vi "Create.vi"(8 "error in (no error)":errorcluster) -> (0 "error out":errorcluster, 3 "BL-Retract-Cmd.lvclass":refnum<class "BL-Retract-Cmd.lvclass">)   [LabVIEW 2013, in "BL-Retract-Cmd.lvclass"]
uses:
  BL-Retract-Cmd.lvclass
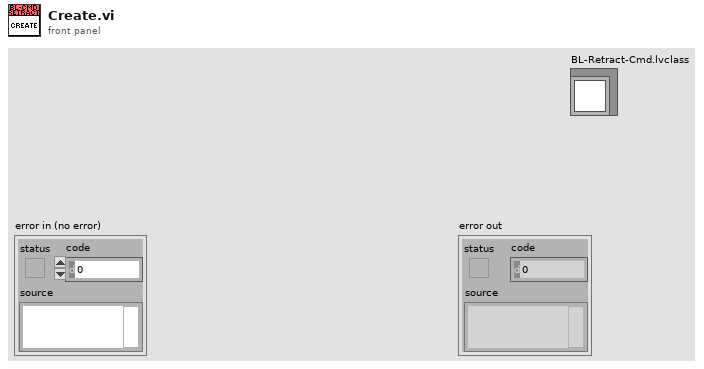
[diagram p1: front panel]
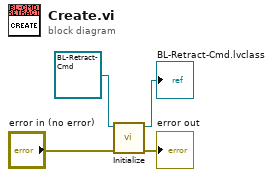
[diagram p0: block diagram]
diagram:
  n1 = call-dynamic "Initialize.vi"("error in (no error)"="error in (no error)", "BL-Retract-Cmd in"=refnum<class "BL-Retract-Cmd.lvclass"> refnum ("BL-Retract-Cmd.lvclass")) -> ("error out"=→"error out":errorcluster, "BL-Retract-Cmd out"=→"BL-Retract-Cmd.lvclass":refnum<class "BL-Retract-Cmd.lvclass">)  [unwired: 8 in]
